vi "Initialize.vi"(8 "error in (no error)":errorcluster, 11 "recent user file":path) -> (0 "error out":errorcluster, 3 "[Data] Recent User out":refnum<class "[Data] Recent User.lvclass">)   [LabVIEW 2020, in "[Data] Recent User.lvclass"]
uses:
  [Data] Recent User.lvclass
  [Data] Recent User.lvclass/[Data] Recent User.ctl
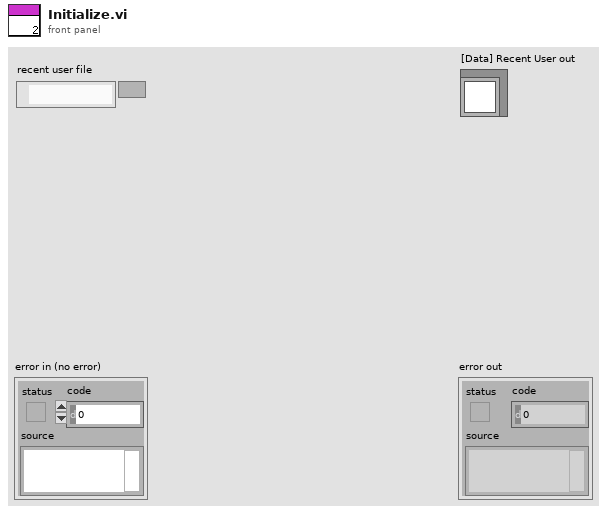
[diagram p1: front panel]
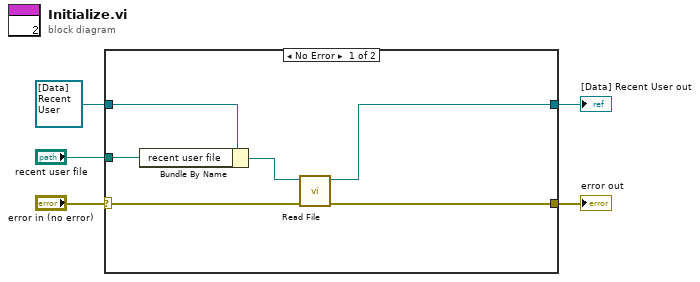
[diagram p0: block diagram]
diagram:
  n1 = case shown="No Error" "error in (no error)" {
    selector: "error in (no error)" -> [w9 w13]
    tunnel: [w6 w13] -> w4
    tunnel: [w7 w12] -> w2
    tunnel: refnum<class "[Data] Recent User.lvclass"> refnum ("[Data] Recent User in") -> [w11 w12]
    tunnel: "recent user file" -> [w10 _]
    frame No Error {
      n2 = Bundle By Name(cluster=w11, "recent user file"=w10) -> (w8:refnum<class "[Data] Recent User.lvclass">)
      n3 = call "Read File.vi"("error in (no error)"=w9, "[Data] Recent User in"=w8) -> ("error out"=w6:errorcluster, "[Data] Recent User out"=w7:refnum<class "[Data] Recent User.lvclass">)  [unwired: 8 in]
    }
    frame Error {
    }
  }
  "error out" <- w4
  "[Data] Recent User out" <- w2
